vi "dataset.add.request.vi"(8 "error in":errorcluster, 9 "Series Tags":map{string, string}(c390), 10 "dataset":refnum<class "dataset.lvclass">, 11 "DataScope Name":string="default") -> (0 "error out":errorcluster, 3 "Request":string)   [LabVIEW 2020, in "asset.lvclass"]
uses:
  asset.lvclass
  datasources/dataset/dataset.lvclass
  datasources/dataset/dataset.lvclass/dataset.ctl
  d09293c4-a5fb-4d14-8e4d-efc786611564.vi
  dbf372a7-e192-454a-a0bf-8f356cd897b9.vi
  datasources/dataset/rid.get.vi
  <vilib>/JDP Science/JSONtext/Variant to JSON Text.vi
  <vilib>/JDP Science/JSONtext/LVClass Serializer/JSONtext LVClass Serializer.lvclass
  nominal types/properties/properties.lvclass
  asset.lvclass/asset.ctl
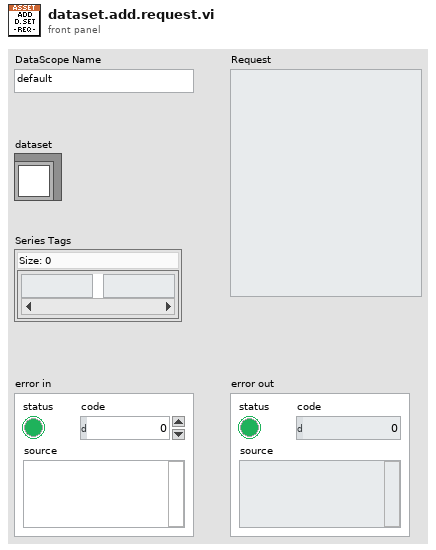
[diagram p1: front panel]
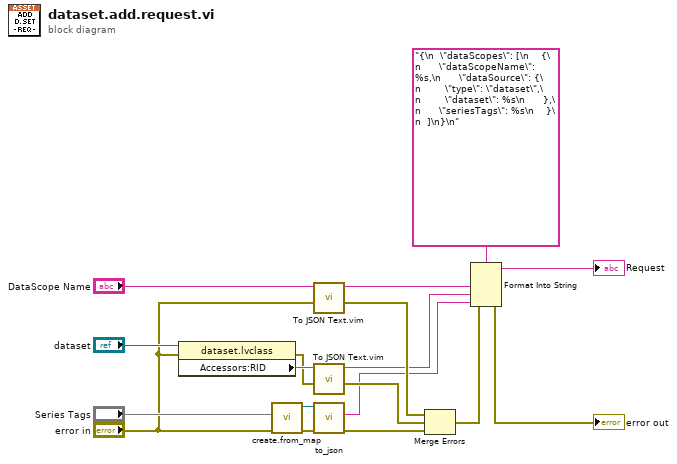
[diagram p0: block diagram]
diagram:
  n1 = property class="dataset.lvclass"(reference="dataset", error in="error in") -> (error out=w2:errorcluster, "Accessors:RID"=w3:string)  [unwired: 1 out]
  n2 = call "create.from_map.vi"("error in"="error in", "properties"="Series Tags") -> ("error out"=w15:errorcluster, "properties out"=w16:refnum<class "properties.lvclass">)  [unwired: 8 in]
  n3 = call "To JSON Text.vim"("error in (no error)"="error in", "Anything"="DataScope Name") -> ("error out"=w18:errorcluster, "<JSON>"=w10:string)  [unwired: 8 in]
  n4 = call "To JSON Text.vim"("error in (no error)"=w2, "Anything"=w3) -> ("error out"=w17:errorcluster, "<JSON>"=w9:string)  [unwired: 8 in]
  n5 = call-dynamic "to_json.vi"("error in"=w15, "properties in"=w16) -> ("error out"=w12:errorcluster, "json"=w8:string)  [unwired: 6 in, 2 out]
  n6 = Merge Errors(w18, w17, w12) -> (w7:errorcluster)
  n7 = Format Into String(format string="{\n  \"dataScopes\": [\n    {\n      \"dataScopeName\": %s,\n      \"dataSource\": {\n        \"type\": \"dataset\",\n        \"dataset\": %s\n      },\n      \"seriesTags\": %s\n    }\n  ]\n}\n", error in=w7, w10, w9, w8) -> (resulting string=→"Request":string, error out=→"error out":errorcluster)  [unwired: 1 in]
